vi "Read Field.vi"(8 "error in (no error)":errorcluster, 11 "Magna Power in":refnum<class "Magna Power.lvclass">) -> (0 "error out":errorcluster, 1 "Current":dbl, 2 "Field (T)":dbl format="%_6f", 3 "Magna Power out":refnum<class "Magna Power.lvclass">, 4 "Voltage":dbl)   [LabVIEW 2023, in "Magna Power.lvclass"]
doc: "Field: Can be positive OR negative, depending on orientation.\n\nRead Field also writes over the object properties of voltage, current, and field. This VI interfaces with both the power supply and the Fluke to do this."
uses:
  Magna Power.lvclass
  Magna Power.lvclass/Magna Power.ctl
  Magna Power Constants.vi
  <vilib>/gmath/NI_Gmath.lvlib
  Fluke Multimeter/Fluke Multimeter.lvclass
panel:
  out "Voltage":string
  out "Current":string
  out "Fluke Voltage (V)":dbl format="%.6f"
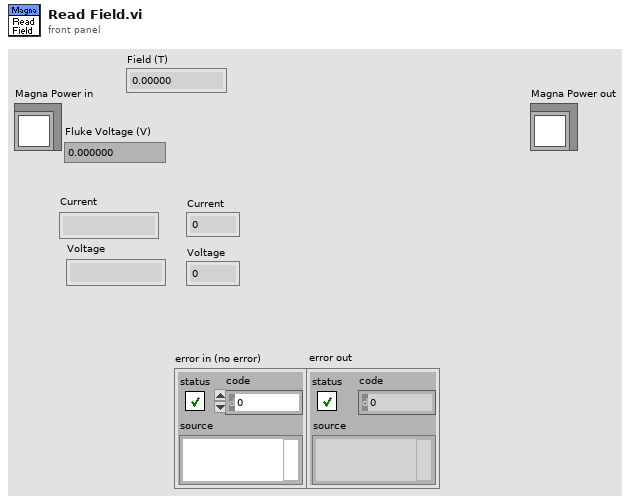
[diagram p1: front panel]
types:
  T1 = cluster{"Magna Current":dbl[], "Magnetic Field":dbl[], "Fluke Voltage":dbl[]}
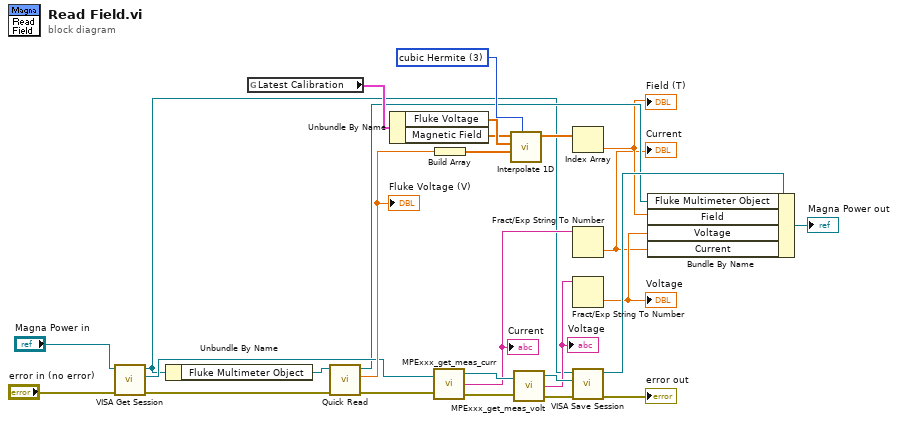
[diagram p0: block diagram]
diagram:
  w21 = 3 items=["nearest", "linear", "spline", "cubic Hermite", "Lagrange"] ("method")
  n1 = call-dynamic "VISA Get Session.vi"("error in (no error)"="error in (no error)", "Instrument.lvclass in"="Magna Power in") -> ("error out"=w16:errorcluster, "VISA Resource Name"=w15:refnum<visa-resource-name>, "Instrument.lvclass out"=w3:refnum<class "Magna Power.lvclass">)  [unwired: 6 in, 1 out]
  n2 = Unbundle By Name(w3) -> ("Fluke Multimeter Object"=w13:refnum<class "Fluke Multimeter.lvclass">)
  n3 = global read "Magna Power Constants.vi" "Latest Calibration"() -> (w27:T1)
  n4 = call "Quick Read.vi"("error in (no error)"=w16, "Fluke Multimeter.lvclass In"=w13) -> ("error out"=w20:errorcluster, "measurement"=w24:dbl, "Fluke Multimeter.lvclass Out"=w8:refnum<class "Fluke Multimeter.lvclass">)  [unwired: 6 in, 1 out]
  "Fluke Voltage (V)" <- w24
  n5 = Unbundle By Name(w27) -> ("Fluke Voltage"=w26:dbl[], "Magnetic Field"=w25:dbl[])
  n6 = call "MPExxx_get_meas_curr.vi"("VISA session"=w15, "error in (no error)"=w20) -> ("dup VISA session"=w18:refnum<visa-resource-name>, "Output Current"=w4:string, "error out"=w19:errorcluster)
  "Current" <- w4
  n7 = Build Array(w24) -> (w23:dbl[])
  n8 = call <vilib>:"Interpolate 1D.vi"("method"=w21, "xi"=w23, "X"=w26, "Y"=w25) -> ("yi"=w22:dbl[])  [unwired: 5 in, 2 out]
  n9 = call "MPExxx_get_meas_volt.vi"("VISA session"=w18, "error in (no error)"=w19) -> ("dup VISA session"=w12:refnum<visa-resource-name>, "Output Voltage"=w5:string, "error out"=w11:errorcluster)
  "Voltage" <- w5
  n10 = Index Array(array=w22) -> (element=w7:dbl)  [unwired: 1 in]
  "Field (T)" <- w7
  n11 = Fract/Exp String To Number(string=w4) -> (number=w1:dbl)  [unwired: 3 in, 1 out]
  "Current" <- w1
  n12 = Fract/Exp String To Number(string=w5) -> (number=w2:dbl)  [unwired: 3 in, 1 out]
  "Voltage" <- w2
  n13 = call-dynamic "VISA Save Session.vi"("error in (no error)"=w11, "VISA Resource Name"=w12, "Instrument.lvclass in"=w3) -> ("error out"=→"error out":errorcluster, "Instrument.lvclass out"=w9:refnum<class "Magna Power.lvclass">)  [unwired: 7 in]
  n14 = Bundle By Name(cluster=w9, "Fluke Multimeter Object"=w8, "Field"=w7, "Voltage"=w2, "Current"=w1) -> (→"Magna Power out":refnum<class "Magna Power.lvclass">)
